vi "Feet per second to Ticks per second.vi"(11 "Drive Velocities (ft/s)":T1) -> (3 "Drive Velocities (ticks/ds)":T1)   [LabVIEW 2020]
doc: "converts feet per second to ticks per decisecond (falcon units)"
uses:
  2023 Charged Up Robot Project/Framework/Robot Global Data.vi
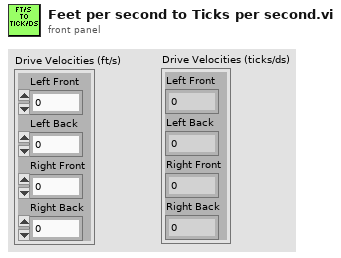
[diagram p1: front panel]
types:
  T1 = cluster{"Left Front":dbl, "Left Back":dbl, "Right Front":dbl, "Right Back":dbl}
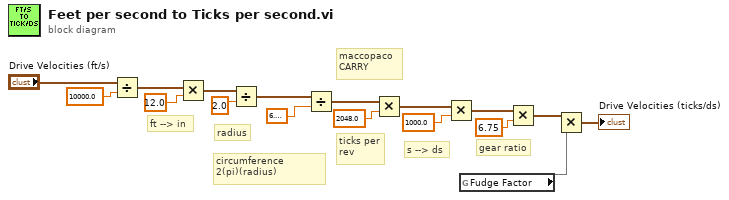
[diagram p0: block diagram]
diagram:
  # "s --> ds"
  # "circumference\n2(pi)(radius)"
  # "ticks per\nrev"
  # "ft --> in"
  # "radius"
  # "gear ratio"
  # "maccopaco\nCARRY"
  n1 = Divide(x="Drive Velocities (ft/s)", y=10000.0) -> (x/y=w16:T1)
  n2 = Multiply(x=w16, y=12.0) -> (x*y=w14:T1)
  n3 = Divide(x=w14, y=2.0) -> (x/y=w12:T1)
  n4 = Divide(x=w12, y=6.283185307179586) -> (x/y=w11:T1)
  n5 = Multiply(x=w11, y=2048.0) -> (x*y=w9:T1)
  n6 = Multiply(x=w9, y=1000.0) -> (x*y=w7:T1)
  n7 = global read "Robot Global Data.vi" "Fudge Factor"() -> (w2)
  n8 = Multiply(x=w7, y=6.75) -> (x*y=w3:T1)
  n9 = Multiply(x=w3, y=w2) -> (x*y=→"Drive Velocities (ticks/ds)":T1)
